vi "Configure Arbitrary Waveform.vi"(7 "Waveform Generator Number (1: Waveform Generator 1)":i32(ring)=1 items=["Waveform Generator 1"=1, "Waveform Generator 2"=2], 8 "error in (no error)":errorcluster, 9 "Enable Interpolation (F: Disable)":bool, 10 "Byte Order (1: LSBF)":i32(ring)=1 items=["MSBF", "LSBF"], 11 "VISA resource name":refnum<visa-resource-name>) -> (0 "error out":errorcluster, 3 "VISA resource name out":refnum<visa-resource-name>)   [LabVIEW 2010, in "Agilent 2000 3000 X-Series.lvlib"]
doc: "Configures the arbitrary waveform generator options."
uses:
  <instrlib>/Agilent 2000 3000 X-Series/Agilent 2000 3000 X-Series.lvlib
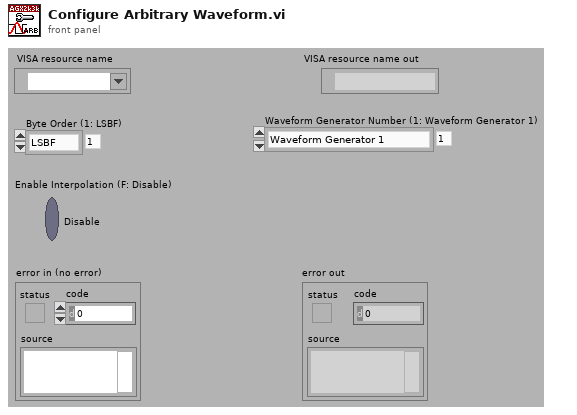
[diagram p1: front panel]
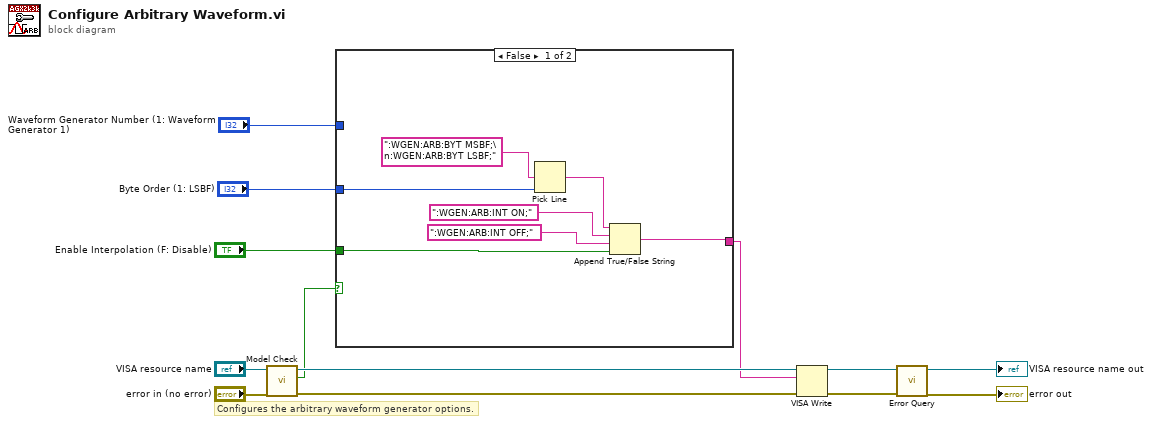
[diagram p0: block diagram]
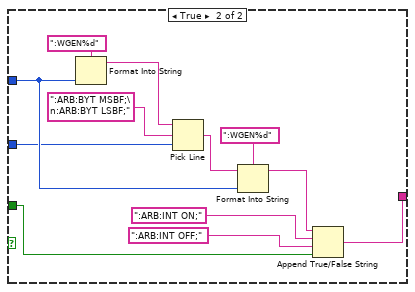
[diagram p2: hidden frame]
diagram:
  # "Configures the arbitrary waveform generator options."
  n1 = call <instrlib>:"Model Check.vi"("error in (no error)"="error in (no error)", "VISA resource name"="VISA resource name") -> ("error out"=w6:errorcluster, "Is 4000 Series"=w3:bool, "VISA resource name out"=w7:refnum<visa-resource-name>)  [unwired: 7 out]
  n2 = case shown="False" w3 {
    tunnel: "Byte Order (1: LSBF)" -> [w16 w21]
    tunnel: "Enable Interpolation (F: Disable)" -> [w15 w22]
    tunnel: [w14 w23] -> w1
    tunnel: "Waveform Generator Number (1: Waveform Generator 1)" -> [_ w25]
    frame False {
      n3 = Pick Line(multi-line string=":WGEN:ARB:BYT MSBF;\n:WGEN:ARB:BYT LSBF;", line index=w16) -> (output string=w19:string)  [unwired: 1 out]
      n4 = Append True/False String(1:w15, 2:":WGEN:ARB:INT OFF;", 3:":WGEN:ARB:INT ON;", 4:w19) -> (0:w14:string)
    }
    frame True {
      n5 = Format Into String(format string=":WGEN%d", w25) -> (resulting string=w28:string)  [unwired: 2 in, 1 out]
      n6 = Pick Line(string ("")=w28, multi-line string=":ARB:BYT MSBF;\n:ARB:BYT LSBF;", line index=w21) -> (output string=w26:string)
      n7 = Format Into String(format string=":WGEN%d", initial string=w26, w25) -> (resulting string=w24:string)  [unwired: 1 in, 1 out]
      n8 = Append True/False String(1:w22, 2:":ARB:INT OFF;", 3:":ARB:INT ON;", 4:w24) -> (0:w23:string)
    }
  }
  n9 = VISA Write(VISA resource name=w7, write buffer=w1, error in (no error)=w6) -> (VISA resource name out=w13:refnum<visa-resource-name>, error out=w12:errorcluster)  [unwired: 1 out]
  n10 = call <instrlib>:"Error Query.vi"("error in (no error)"=w12, "VISA resource name"=w13) -> ("error out"=→"error out":errorcluster, "VISA resource name out"=→"VISA resource name out":refnum<visa-resource-name>)  [unwired: 8 out]
